vi "Do.vi"(8 "error in (no error)":errorcluster, 9 "CommandQueueIn":refnum<queue>, 10 "DataNotifierIn":refnum<notifier>, 11 "CommandCopy in":refnum<class "Measurement.lvclass">) -> (0 "error out":errorcluster, 1 "ExitFlag":bool, 2 "DataNotifierOut":refnum<notifier>, 3 "CommandCopy out":refnum<class "Measurement.lvclass">)   [LabVIEW 2013, in "Measurement.lvclass"]
uses:
  Measurement.lvclass
  SystemData.lvclass/SystemData.lvclass
  RootCommand.lvclass/RootCommand.lvclass
  Display.lvclass/Display.lvclass
  SystemData.lvclass/SystemData.lvclass/SystemData.ctl
  Generator.lvclass/Generator.lvclass
panel:
  # "notifier包裝SystemData物件的參考"
  # "命令物件序列參考"
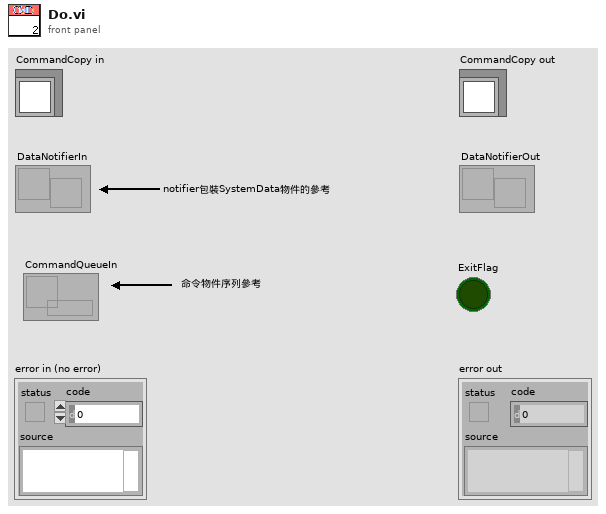
[diagram p1: front panel]
types:
  T1 = typedef "SystemData.lvclass/SystemDataTypeDefine.ctl" = cluster{"ThisVIParameter":cluster{"ThisVIPath":path, "ThisVIReference":refnum<vi>, "AllControlReference":refnum<vi>[]}, "GeneratorParameter":cluster{"Frequency":dbl, "Amplitude":dbl}, "WaveformBuffer":waveform(dbl), "SourceSelect":u16, "GeneratorClassArray":refnum<class "Generator.lvclass">[]}
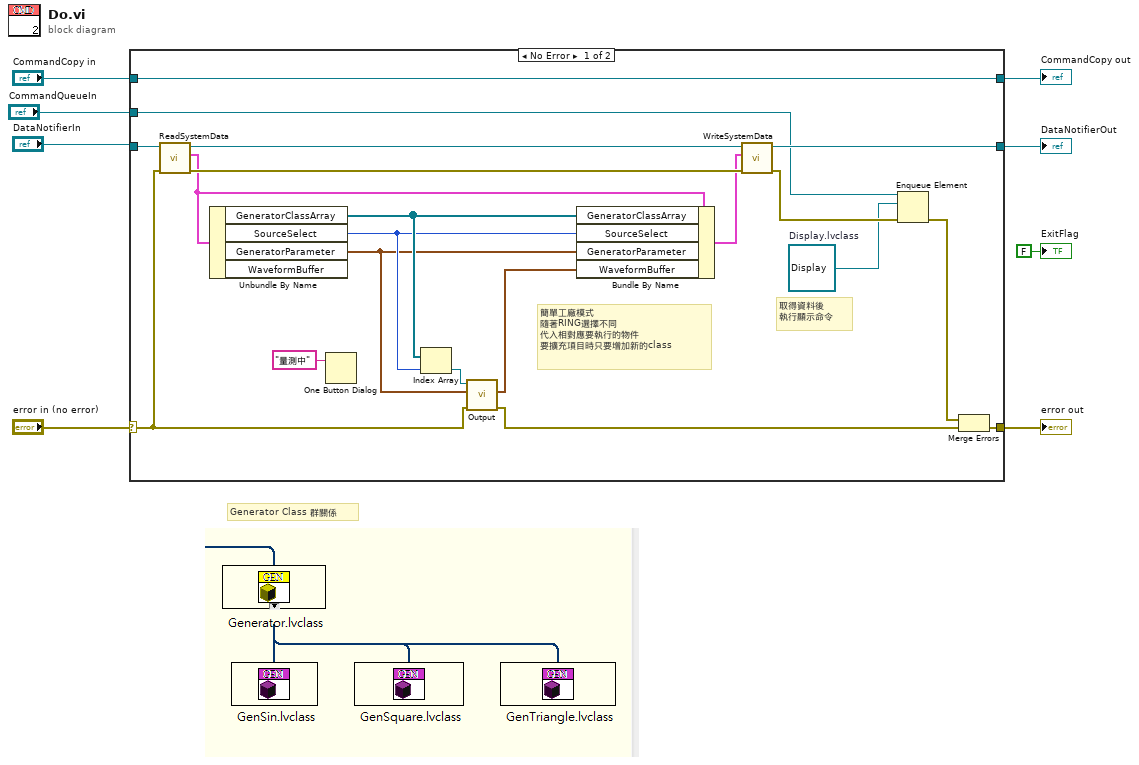
[diagram p0: block diagram]
diagram:
  # "Generator Class 群關係"
  n1 = case shown="No Error" "error in (no error)" {
    selector: "error in (no error)" -> [w19 w31]
    tunnel: [w18 w31] -> w4
    tunnel: [w28 w30] -> w3
    tunnel: "CommandCopy in" -> [w28 w30]
    tunnel: "DataNotifierIn" -> [w27 w29]
    tunnel: [w22 w29] -> w2
    tunnel: "CommandQueueIn" -> [w21 _]
    frame No Error {
      w15 = refnum<class "Display.lvclass"> refnum  # Display.lvclass
      # "簡單工廠模式\n隨著RING選擇不同\n代入相對應要執行的物件\n要擴充項目時只要增加新的class"
      # "取得資料後\n執行顯示命令"
      n2 = call "ReadSystemData.vi"("error in (no error)"=w19, "DataNotifierIn"=w27) -> ("error out"=w25:errorcluster, "SystemData"=w24:T1, "DataNotifierIn"=w26:refnum<notifier>)  [unwired: 7 in]
      n3 = Unbundle By Name(w24) -> ("GeneratorClassArray"=w14:refnum<class "Generator.lvclass">[], "SourceSelect"=w13:u16, "GeneratorParameter"=w10:cluster{"Frequency":dbl, "Amplitude":dbl})  [unwired: 1 out]
      n4 = One Button Dialog(message="量測中") -> ()  [unwired: 1 in, 1 out]
      n5 = Index Array(array=w14, index=w13) -> (element=w12:refnum<class "Generator.lvclass">)
      n6 = call-dynamic "Output.vi"("error in (no error)"=w19, "SignalGeneratorParameter"=w10, "Generator in"=w12) -> ("error out"=w16:errorcluster, "Waveform"=w11:waveform(dbl))  [unwired: 6 in, 1 out]
      n7 = Bundle By Name(cluster=w24, "GeneratorClassArray"=w14, "SourceSelect"=w13, "GeneratorParameter"=w10, "WaveformBuffer"=w11) -> (w23:T1)
      n8 = call "WriteSystemData.vi"("error in (no error)"=w25, "SystemData"=w23, "DataNotifierIn"=w26) -> ("error out"=w20:errorcluster, "DataNotifierOut"=w22:refnum<notifier>)  [unwired: 7 in]
      n9 = Enqueue Element(queue=w21, element=w15, error in (no error)=w20) -> (error out=w17:errorcluster)  [unwired: 1 in, 2 out]
      n10 = Merge Errors(w17, w16) -> (w18:errorcluster)
    }
    frame Error {
    }
  }
  "error out" <- w4
  "CommandCopy out" <- w3
  "DataNotifierOut" <- w2
  "ExitFlag" <- FALSE ("ExitFlag")
